vi "Print Report.vi"(0 "report in":refnum<class "NI_Word.lvclass">, 5 "printer name (default)":string, 9 "number of copies (1)":i32=1, 11 "error in (no error)":errorcluster) -> (4 "report out":refnum<class "NI_Word.lvclass">, 15 "error out":errorcluster)   [LabVIEW 2015, in "NI_Word.lvclass"]
doc: "Prints a report to a designated printer or to the default printer on the computer."
uses:
  <vilib>/Utility/NIReport.llb/Word/NI_Word.lvclass
  <vilib>/Utility/NIReport.llb/Word/NI_Word.lvclass/NI_Word.ctl
  <vilib>/addons/_office/NI_ReportGenerationToolkit.lvlib
  <vilib>/Utility/NIReport.llb/NI_ReportGenerationCore.lvlib
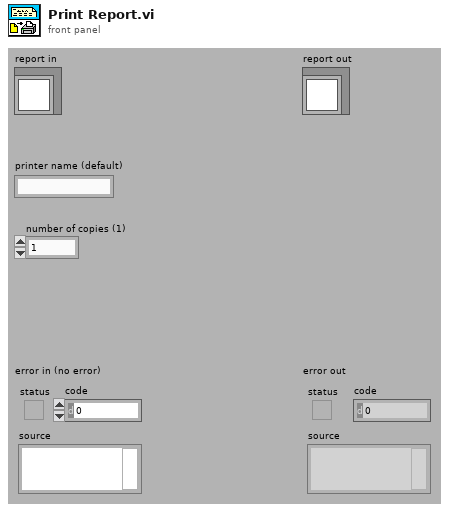
[diagram p1: front panel]
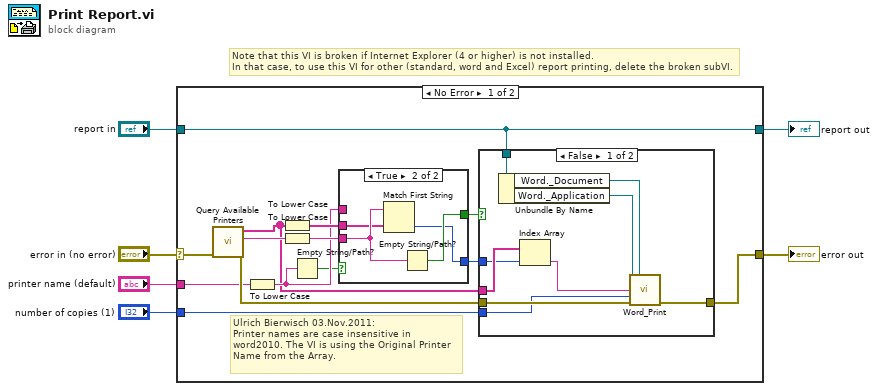
[diagram p0: block diagram]
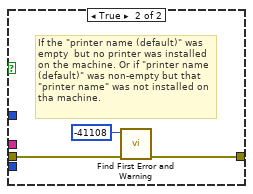
[diagram p2: hidden frame]
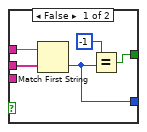
[diagram p3: hidden frame]
diagram:
  # "Note that this VI is broken if Internet Explorer (4 or higher) is not installed.\nIn that case, to use this VI for other (standard, word and Excel) report printing, delete the broken subVI."
  n1 = case shown="No Error" "error in (no error)" {
    selector: "error in (no error)" -> [w14 w43]
    tunnel: [w10 w43] -> w5
    tunnel: [w12 w42] -> w3
    tunnel: "report in" -> [w12 w42]
    tunnel: "printer name (default)" -> [w7 _]
    tunnel: "number of copies (1)" -> [w11 _]
    frame No Error {
      # "Ulrich Bierwisch 03.Nov.2011:\nPrinter names are case insensitive in word2010. The VI is using the Original Printer Name from the Array."
      n2 = call <vilib>:"Query Available Printers.vi"("error in (no error)"=w14) -> ("error out"=w13:errorcluster, "default printer"=w17:string, "system configured printers"=w9:string[])  [unwired: 8 out]
      n3 = To Lower Case(string=w7) -> (all lower case string=w18:string)
      n4 = To Lower Case(string=w9) -> (all lower case string=w19:string[])
      n5 = To Lower Case(string=w17) -> (all lower case string=w20:string)
      n6 = Empty String/Path?(string/path=w18) -> (empty?=w15:bool)
      n7 = case shown="True" w15 {
        tunnel: w18 -> [w34 _]
        tunnel: [w35 w41] -> w16
        tunnel: w19 -> [w36 w39]
        tunnel: w20 -> [_ w40]
        tunnel: [w33 w38] -> w8
        frame False {
          n8 = Match First String(2:w36, 3:w34) -> (0:w33:i32)  [unwired: 1 out]
          n9 = Equal?(x=-1 ("y"), y=w33) -> (x = y?=w35:bool)
        }
        frame True {
          n10 = Match First String(2:w39, 3:w40) -> (0:w38:i32)  [unwired: 1 out]
          n11 = Empty String/Path?(string/path=w40) -> (empty?=w41:bool)
        }
      }
      n12 = case shown="False" w16 {
        tunnel: w9 -> [w23 _]
        tunnel: w13 -> [w27 w31]
        tunnel: w12 -> [w26 _]
        tunnel: w11 -> [w25 _]
        tunnel: [w24 w30] -> w10
        tunnel: w8 -> [w22 _]
        frame False {
          n13 = Unbundle By Name(w26) -> ("Word._Document"=w28:refnum<k7>, "Word._Application"=w29:refnum<k7>)
          n14 = Index Array(array=w23, index=w22) -> (element=w21:string)
          n15 = call <vilib>:"Word_Print.vi"("Word._Application"=w29, "Word._Document"=w28, "printer name (default)"=w21, "number of copies (1)"=w25, "error in (no error)"=w27) -> ("error out"=w24:errorcluster)  [unwired: 10 out]
        }
        frame True {
          # "If the \"printer name (default)\" was empty  but no printer was installed on the machine. Or if \"printer name (default)\" was non-empty but that \"printer name\" was not installed on tha machine."
          n16 = call <vilib>:"Find First Error and Warning.vi"("error in (no error)"=w31, "error code"=-41108) -> ("error out"=w30:errorcluster)  [unwired: 5 out]
        }
      }
    }
    frame Error {
    }
  }
  "error out" <- w5
  "report out" <- w3
